vi "Create System Output Limits.vi"(8 "error in (no error)":errorcluster, 11 "Device Item Ref in":T1 format="%.0x") -> (0 "error out":errorcluster)   [LabVIEW 2020, in "G5 Regatron Custom Device System Explorer.lvlib"]
uses:
  G5 Regatron Custom Device System Explorer.lvlib
  <vilib>/NI VeriStand/Custom Device API/Custom Device Channel Type.ctl
  <vilib>/NI VeriStand/Custom Device API/Custom Device API.lvlib
  <vilib>/NI VeriStand/Custom Device API/Custom Device Channel.ctl
  <vilib>/NI VeriStand/Custom Device API/Custom Device Item Ref.ctl
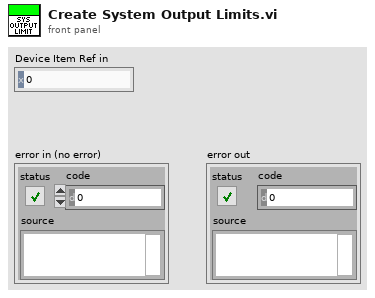
[diagram p1: front panel]
types:
  T1 = typedef "Custom Device API.lvlib/Custom Device Item Ref.ctl" = u64
  T2 = typedef "Custom Device API.lvlib/Custom Device Channel.ctl" = cluster{"Type":T3, "Units":string, "Default Value":dbl, "Faultable":bool, "Scalable":bool}
  T3 = typedef "Custom Device API.lvlib/Custom Device Channel Type.ctl" = enum16{"Input", "Output"}
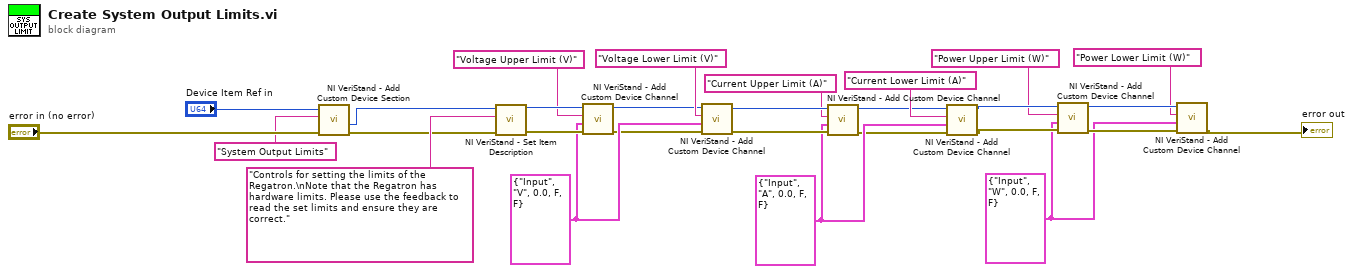
[diagram p0: block diagram]
diagram:
  w15 = T2 {"Type"=enum."Input", "Units"="W", "Default Value"=0.0, "Faultable"=FALSE, "Scalable"=FALSE} ("Channel")
  w12 = T2 {"Type"=enum."Input", "Units"="V", "Default Value"=0.0, "Faultable"=FALSE, "Scalable"=FALSE} ("Channel")
  w5 = T2 {"Type"=enum."Input", "Units"="A", "Default Value"=0.0, "Faultable"=FALSE, "Scalable"=FALSE} ("Channel")
  n1 = call <vilib>:"NI VeriStand - Add Custom Device Section.vi"("error in (no error)"="error in (no error)", "Section Name"="System Output Limits", "Parent Ref in"="Device Item Ref in") -> ("error out"=w24:errorcluster, "Section Ptr"=w26:T1)  [unwired: 5 in, 2 out]
  n2 = call <vilib>:"NI VeriStand - Set Item Description.vi"("error in (no error)"=w24, "Description"="Controls for setting the limits of the Regatron.\nNote that the Regatron has hardware limits. Please use the feedback to read the set limits and ensure they are correct.", "Item Ref in"=w26) -> ("error out"=w25:errorcluster, "Item Ref out"=w27:T1)  [unwired: 6 in, 1 out]
  n3 = call <vilib>:"NI VeriStand - Add Custom Device Channel.vi"("error in (no error)"=w25, "Channel"=w12, "Channel Name"="Voltage Upper Limit (V)", "Parent Ref in"=w27) -> ("error out"=w9:errorcluster, "Parent Ref out"=w10:T1)  [unwired: 4 in, 2 out]
  n4 = call <vilib>:"NI VeriStand - Add Custom Device Channel.vi"("error in (no error)"=w9, "Channel"=w12, "Channel Name"="Voltage Lower Limit (V)", "Parent Ref in"=w10) -> ("error out"=w14:errorcluster, "Parent Ref out"=w13:T1)  [unwired: 4 in, 2 out]
  n5 = call <vilib>:"NI VeriStand - Add Custom Device Channel.vi"("error in (no error)"=w14, "Channel"=w5, "Channel Name"="Current Upper Limit (A)", "Parent Ref in"=w13) -> ("error out"=w2:errorcluster, "Parent Ref out"=w3:T1)  [unwired: 4 in, 2 out]
  n6 = call <vilib>:"NI VeriStand - Add Custom Device Channel.vi"("error in (no error)"=w2, "Channel"=w5, "Channel Name"="Current Lower Limit (A)", "Parent Ref in"=w3) -> ("error out"=w21:errorcluster, "Parent Ref out"=w20:T1)  [unwired: 4 in, 2 out]
  n7 = call <vilib>:"NI VeriStand - Add Custom Device Channel.vi"("error in (no error)"=w21, "Channel"=w15, "Channel Name"="Power Upper Limit (W)", "Parent Ref in"=w20) -> ("error out"=w18:errorcluster, "Parent Ref out"=w17:T1)  [unwired: 4 in, 2 out]
  n8 = call <vilib>:"NI VeriStand - Add Custom Device Channel.vi"("error in (no error)"=w18, "Channel"=w15, "Channel Name"="Power Lower Limit (W)", "Parent Ref in"=w17) -> ("error out"=→"error out":errorcluster)  [unwired: 4 in, 3 out]
